vi "Timing_FGV.vi"(7 "Task":enum16{"Reset", "Run", "Pause"}(ring), 8 "error in (no error)":errorcluster, 11 "Time Period (s)":u32=5) -> (0 "error out":errorcluster, 2 "Period Done":bool, 3 "Elapsed Time":dbl)   [LabVIEW 2020]
doc: "FGV that keeps track of station timing. The pause task will halt a current time keeping and must be run immediately before resuming timing."
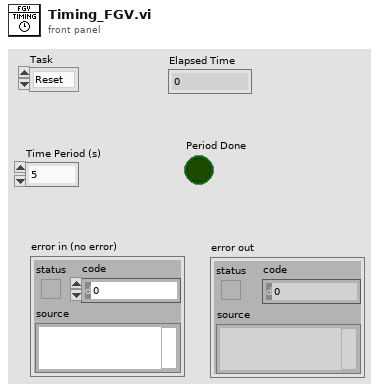
[diagram p1: front panel]
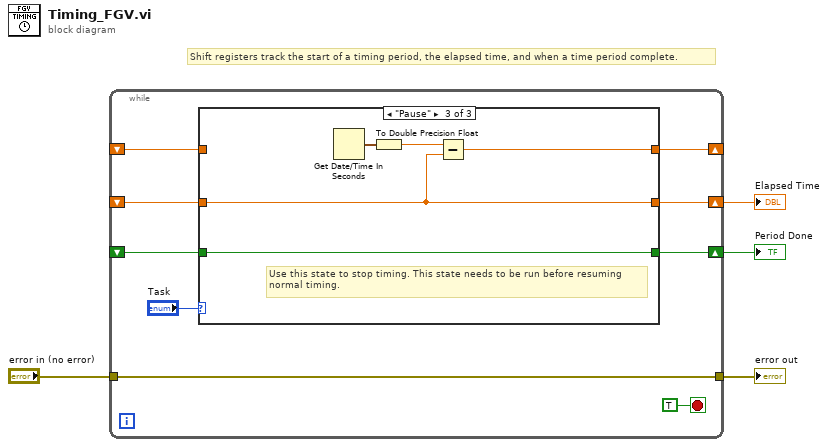
[diagram p0: block diagram]
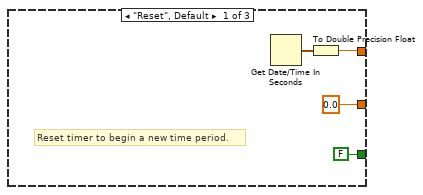
[diagram p2: hidden frame]
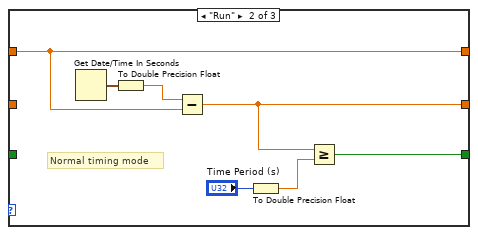
[diagram p3: hidden frame]
diagram:
  # "Shift registers track the start of a timing period, the elapsed time, and when a time period complete."
  n1 = while {
    shift-right: [w11] -> _
    shift-left: _ -> [w9]
    tunnel: "error in (no error)" -> [w7]
    tunnel: [w7] -> w1
    shift-right: [w10] -> w4
    shift-left: _ -> [w5]
    shift-right: [w8] -> w3
    shift-left: _ -> [w6]
    stop <- TRUE stop-if-true
    n2 = case shown="\"Pause\"" "Task" {
      tunnel: [w16 w22 w26] -> w11
      tunnel: [0.0 w19 w25] -> w10
      tunnel: w9 -> [_ w22 _]
      tunnel: [FALSE w18 w29] -> w8
      tunnel: w6 -> [_ _ w29]
      tunnel: w5 -> [_ _ w25]
      frame "Reset", Default {
        # "Reset timer to begin a new time period."
        n3 = Get Date/Time In Seconds() -> (seconds since 1Jan1904=w17:timestamp)
        n4 = To Double Precision Float(number=w17) -> (double precision float=w16:dbl)
      }
      frame "Run" {
        # "Normal timing mode"
        n5 = Get Date/Time In Seconds() -> (seconds since 1Jan1904=w24:timestamp)
        n6 = To Double Precision Float(number=w24) -> (double precision float=w23:dbl)
        n7 = Subtract(x=w23, y=w22) -> (x-y=w19:dbl)
        n8 = To Double Precision Float(number="Time Period (s)") -> (double precision float=w20:dbl)
        n9 = Greater Or Equal?(x=w19, y=w20) -> (x >= y?=w18:bool)
      }
      frame "Pause" {
        # "Use this state to stop timing. This state needs to be run before resuming\nnormal timing."
        n10 = Get Date/Time In Seconds() -> (seconds since 1Jan1904=w28:timestamp)
        n11 = To Double Precision Float(number=w28) -> (double precision float=w27:dbl)
        n12 = Subtract(x=w27, y=w25) -> (x-y=w26:dbl)
      }
    }
  }
  "Elapsed Time" <- w4
  "Period Done" <- w3
  "error out" <- w1
